vi "Asynchronous Launcher - sequenceManagerWorker.vi"(6 "Worker Alias":string="sequenceManagerWkr", 8 "error in":errorcluster, 9 "Initialization Data":T1, 11 "sequenceManagerWorker in":refnum<class "sequenceManagerWorker.lvclass">) -> (0 "error out":errorcluster, 3 "sequenceManagerWorker out":refnum<class "sequenceManagerWorker.lvclass">)   [LabVIEW 2023]
doc: "This VI calls a Worker's Launcher VI asynchronously, and returns the Worker's object containing the Worker's Public Properties. The returned Worker's object can be used with the Worker's Public API Request VIs from applications external to the Workers application (eg. TestStand).\n---"
uses:
  Workers/sequenceManagerWorker/sequenceManagerWorker.lvclass
  Workers/sequenceManagerWorker/Response Cases.ctl
  Workers/sequenceManagerWorker/Initialization Data.ctl
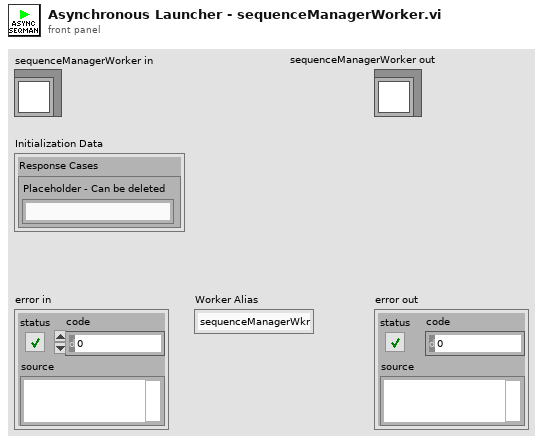
[diagram p1: front panel]
types:
  T1 = typedef "sequenceManagerWorker.lvclass/Initialization Data.ctl" = cluster{"Response Cases":T2}
  T2 = typedef "sequenceManagerWorker.lvclass/Response Cases.ctl" = cluster{"Placeholder - Can be deleted":string}
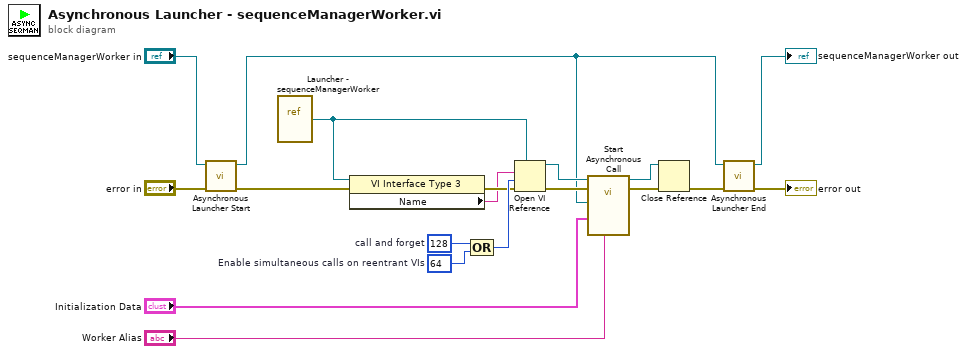
[diagram p0: block diagram]
diagram:
  w18 = 64  # Enable simultaneous calls on reentrant VIs
  w15 = 128  # call and forget
  n1 = call-dynamic "Asynchronous Launcher Start.vi"("error in (no error)"="error in", "Worker in"="sequenceManagerWorker in") -> ("error out"=w19:errorcluster, "Worker out"=w1:refnum<class "sequenceManagerWorker.lvclass">)  [unwired: 8 in]
  n2 = vi-ref "Launcher - sequenceManagerWorker.vi"() -> (w4:refnum<vi>)
  n3 = property class="VI Interface Type 3"(reference=w4, error in=w19) -> (error out=w13:errorcluster, "Name"=w12:string)  [unwired: 1 out]
  n4 = Compound Arithmetic op=OR(w15, w18) -> (w16:i32)
  n5 = Open VI Reference(type specifier VI Refnum (for type only)=w4, vi path=w12, options=w16, error in (no error)=w13) -> (vi reference=w17:refnum<vi>, error out=w11:errorcluster)  [unwired: 2 in]
  n6 = call-by-ref "Start Asynchronous Call"(reference=w17, error in=w11, "Worker Alias"="Worker Alias", "Initialization Data"="Initialization Data", "sequenceManagerWorker in"=w1) -> (reference out=w9:refnum<vi>, error out=w10:errorcluster)  [unwired: 8 in, 1 out]
  n7 = Close Reference(reference=w9, error in (no error)=w10) -> (error out=w14:errorcluster)
  n8 = call-dynamic "Asynchronous Launcher End.vi"("error in (no error)"=w14, "Worker in"=w1) -> ("error out"=→"error out":errorcluster, "Worker out"=→"sequenceManagerWorker out":refnum<class "sequenceManagerWorker.lvclass">)  [unwired: 8 in]
